vi "IHM_GetOngletControlsRefs.vi"(8 "Error In":errorcluster caption="Entrée d'erreur", 10 "PageName":string, 11 "OngletRef":refnum<vi>) -> (0 "Error Out":errorcluster caption="Sortie d'erreur", 2 "CtrlsRefs_OUT":T1[](array[typedef]), 3 "ControlsOnPage":refnum<vi>[](array[refnum]))   [LabVIEW 2013]
uses:
  CTL/CtrlRef.ctl
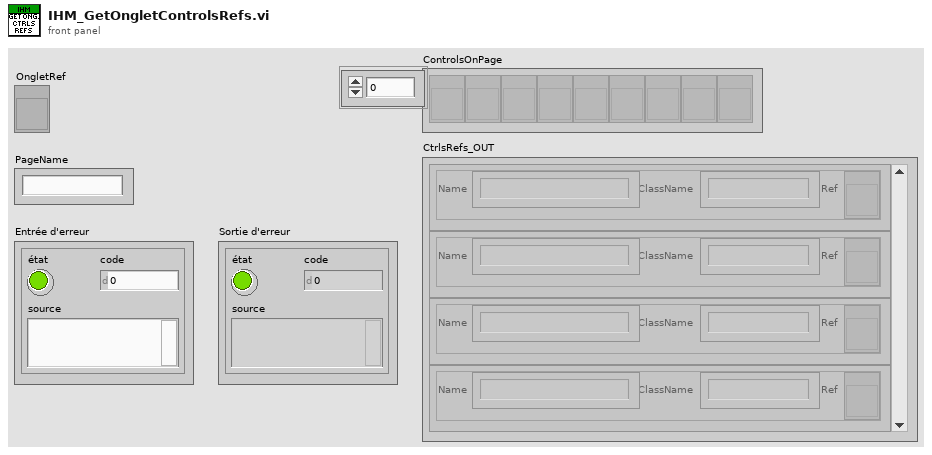
[diagram p1: front panel]
types:
  T1 = typedef "CtrlRef.ctl" = cluster{"Name":string, "Ref":refnum<vi>, "ClassName":string}
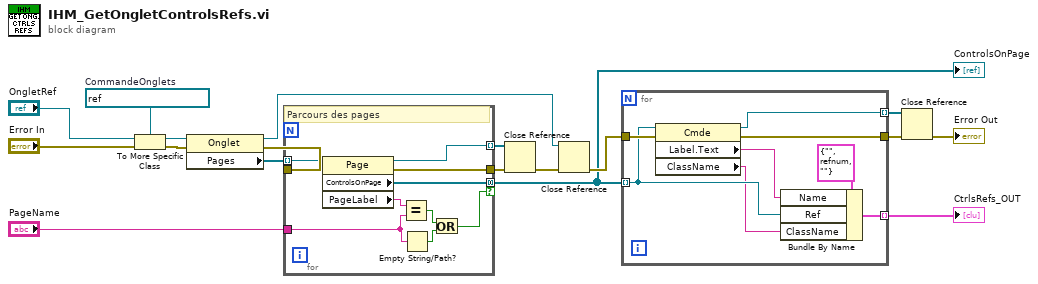
[diagram p0: block diagram]
diagram:
  w10 = refnum<vi> refnum  # CommandeOnglets
  n1 = To More Specific Class(target class=w10, reference="OngletRef", error in="Error In") -> (specific class reference=w8:refnum<vi>, error out=w9:errorcluster)
  n2 = property class="Onglet"(reference=w8, error in=w9) -> (reference out=w13:refnum<vi>, error out=w11:errorcluster, "Pages"=w12:refnum<vi>[])
  n3 = for {
    tunnel: w12 -> [w28] mode=indexing
    tunnel: w11 -> [w27]
    tunnel: [w26] -> w6
    tunnel: [w25] -> w7 mode=indexing
    tunnel: [w24] -> w3 mode=concatenating if=w19
    tunnel: "PageName" -> [w22]
    # "Parcours des pages"
    n4 = property class="Page"(reference=w28, error in=w27) -> (reference out=w25:refnum<vi>, error out=w26:errorcluster, "ControlsOnPage"=w24:refnum<vi>[], "PageLabel"=w23:string)
    n5 = Equal?(x=w23, y=w22) -> (x = y?=w21:bool)
    n6 = Empty String/Path?(string/path=w22) -> (empty?=w20:bool)
    n7 = Or(x=w21, y=w20) -> (x .or. y?=w19:bool)
  }
  "ControlsOnPage" <- w3
  n8 = Close Reference(reference=w7, error in (no error)=w6) -> (error out=w14:errorcluster)
  n9 = Close Reference(reference=w13, error in (no error)=w14) -> (error out=w15:errorcluster)
  n10 = for {
    tunnel: w3 -> [w31] mode=indexing
    tunnel: [w32] -> w18 mode=indexing
    tunnel: w15 -> [w36]
    tunnel: [w35] -> w17
    tunnel: [w34] -> w16 mode=indexing
    n11 = property class="Cmde"(reference=w31, error in=w36) -> (reference out=w34:refnum<vi>, error out=w35:errorcluster, "Label.Text"=w29:string, "ClassName"=w30:string)
    n12 = Bundle By Name(cluster=T1 {"Name"="", "Ref"=refnum, "ClassName"=""} ("CtrlRef"), "Name"=w29, "Ref"=w31, "ClassName"=w30) -> (w32:T1)
  }
  "CtrlsRefs_OUT" <- w18
  n13 = Close Reference(reference=w16, error in (no error)=w17) -> (error out=→"Error Out":errorcluster)
